vi "FGVFileSavePath.vi"(6 "Type":enum16{"Read", "Write"}(ring), 11 "FileSaveParameters":T1) -> (3 "FileSaveParameters":T1)   [LabVIEW 2024]
uses:
  FileSaver/#SaveFileParameters.ctl
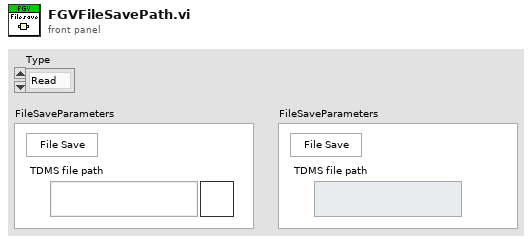
[diagram p1: front panel]
types:
  T1 = typedef "#SaveFileParameters.ctl" = cluster{"StartSaveFile":bool, "TDMS file path":path}
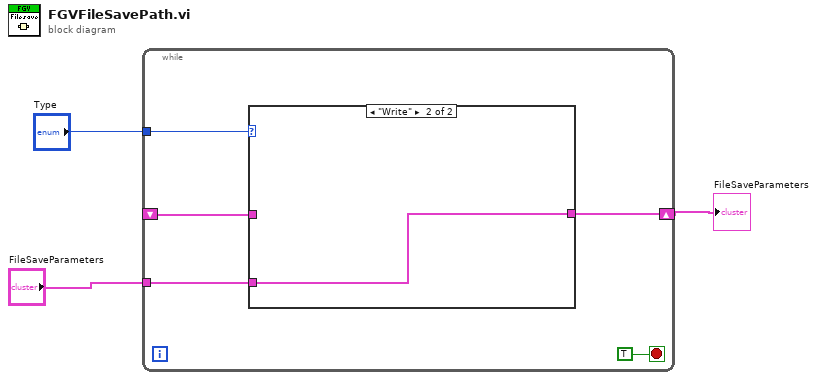
[diagram p0: block diagram]
diagram:
  n1 = while {
    tunnel: "Type" -> [w7]
    shift-right: [w5] -> w1
    shift-left: _ -> [w6]
    tunnel: "FileSaveParameters" -> [w4]
    stop <- TRUE stop-if-true
    n2 = case shown="\"Write\"" w7 {
      tunnel: w6 -> [w9 _]
      tunnel: [w9 w10] -> w5
      tunnel: w4 -> [_ w10]
      frame "Read" {
      }
      frame "Write" {
      }
    }
  }
  "FileSaveParameters" <- w1
